vi "GetOCRResultName.vi"(7 "ProjectName":string="Prj", 8 "error in (no error)":errorcluster, 10 "data":T2, 11 "ROI_Name":string="ROI1") -> (0 "error out":errorcluster, 3 "Array":string[](array[string]))   [LabVIEW 2019]
uses:
  Controls/OCR/Analysis_OCR_Setting Parameter.ctl
  Controls/OCR/Analysis_OCR_Result.ctl
panel:
  in  "Analysis_OCR_Result":T1
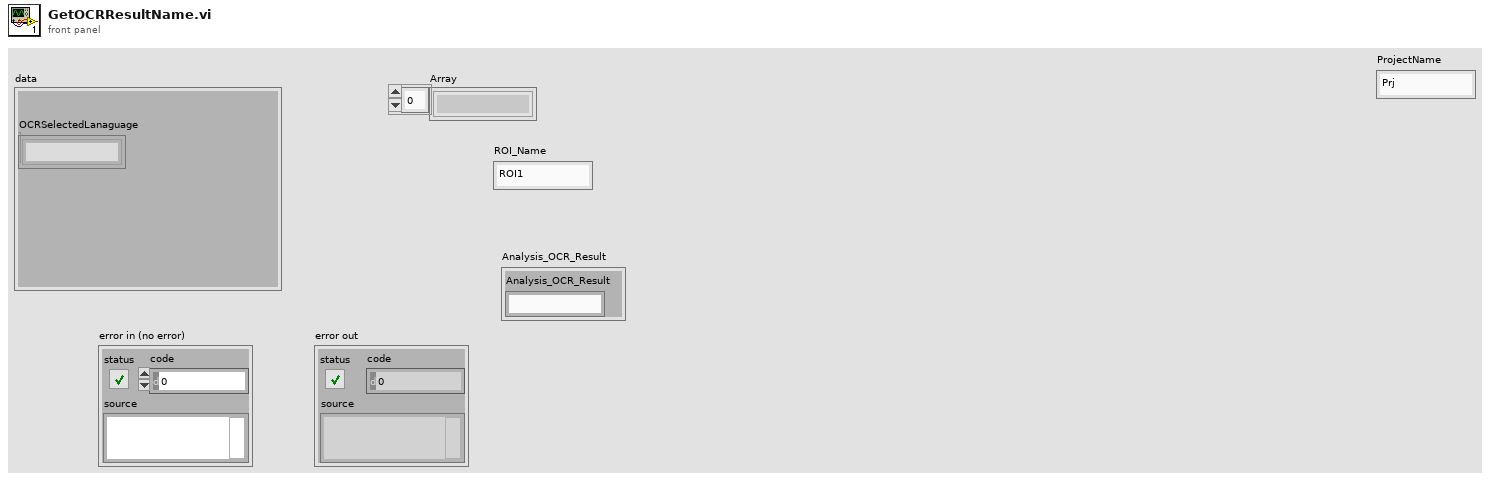
[diagram p1: front panel]
types:
  T1 = typedef "Analysis_OCR_Result.ctl" = cluster{"Analysis_OCR_Result":string}
  T2 = typedef "Analysis_OCR_Setting Parameter.ctl" = cluster{"OCRSelectedLanaguage":string[]}
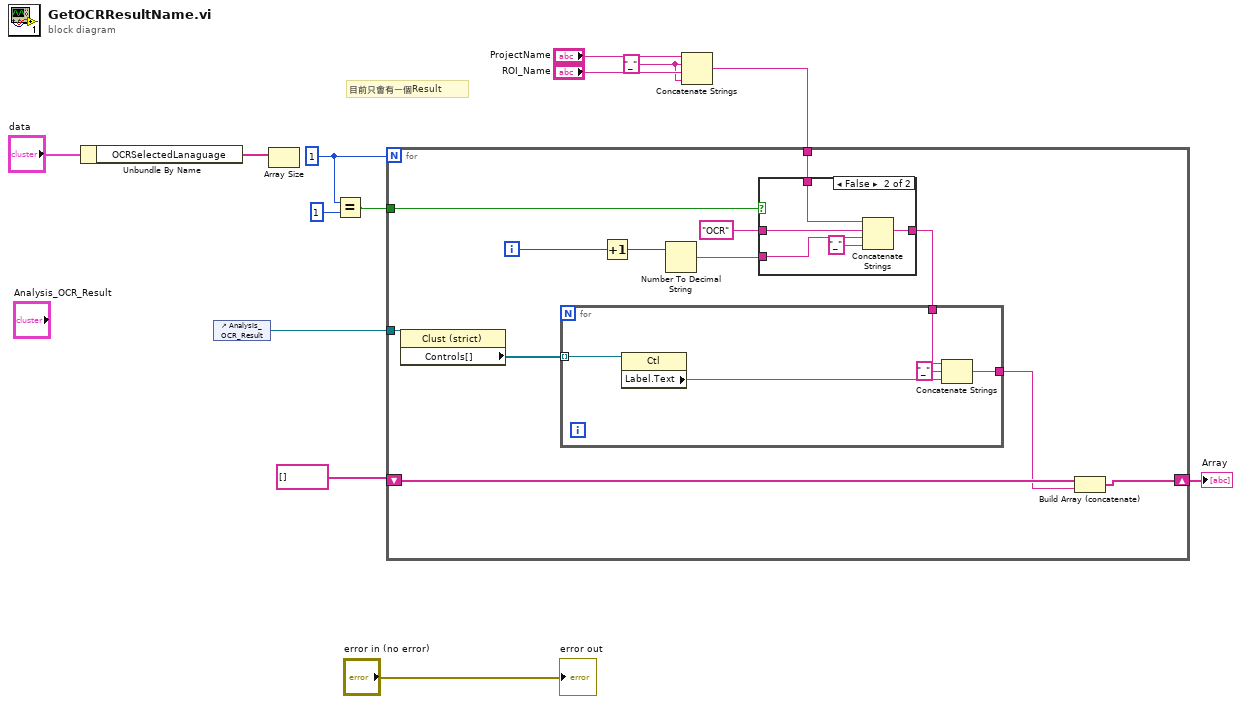
[diagram p0: block diagram]
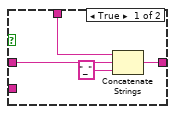
[diagram p2: hidden frame]
diagram:
  w1 = 1
  w8 = "_" ("string")
  # "目前只會有一個Result"
  n1 = Unbundle By Name("data") -> ("OCRSelectedLanaguage"=w12:string[])
  n2 = control-ref of="Analysis_OCR_Result"() -> (w4:refnum<vi>)
  n3 = Array Size(array=w12) -> ()  [unwired: 1 out]
  n4 = Equal?(x=w1, y=1) -> (x = y?=w6:bool)
  n5 = Concatenate Strings("ProjectName", w8, "ROI_Name", w8) -> (w7:string)
  n6 = for {
    N: w1 -> [_]
    tunnel: w7 -> [w21]
    tunnel: w6 -> [w20]
    tunnel: w4 -> [w19]
    shift-right: [w14] -> w2
    shift-left: string[] [] -> [w16]
    i -> [w22]
    n7 = property class="Clust (strict)"(reference=w19) -> ("Controls[]"=w18:refnum<vi>[])  [unwired: 1 in, 2 out]
    n8 = Increment(x=w22) -> (x+1=w25:i32)
    n9 = Number To Decimal String(number=w25) -> (decimal integer string=w24:string)  [unwired: 1 in]
    n10 = case shown="False" w20 {
      tunnel: w21 -> [w34 w39]
      tunnel: w24 -> [_ w37]
      tunnel: [w33 w38] -> w17
      tunnel: "OCR" ("string") -> [w32 w36]
      frame True {
        n11 = Concatenate Strings(w34, w32, "_" ("string")) -> (w33:string)
      }
      frame False {
        n12 = Concatenate Strings(w39, w36, w37, "_" ("string")) -> (w38:string)
      }
    }
    n13 = for {
      tunnel: w18 -> [w30] mode=indexing
      tunnel: w17 -> [w29]
      tunnel: [w26] -> w15
      n14 = property class="Ctl"(reference=w30) -> ("Label.Text"=w27:string)  [unwired: 1 in, 2 out]
      n15 = Concatenate Strings(w29, "_" ("string"), w27) -> (w26:string)
    }
    n16 = Build Array (concatenate)(w16, w15) -> (w14:string[])
  }
  "Array" <- w2
  "error out" <- "error in (no error)"
